vi "Simple UDP - Sender.vi"(8 "Stop":bool, 11 "Hand Coord.":dbl[](array[numeric])=[1000.0, 1000.0, 1000.0]) -> ()   [LabVIEW 2017]
doc: "The UDP protocol differs from TCP in that there is no error-checking with the packets of information that are sent, and thus no guarantee whatsoever that an intended recipient will actually receive a given piece of data.\n\nUDP does offer the ability to \"broadcast\" data across a network--simply specify an IP Address of all ones (255.255.255.255) to attempt to broadcast information network-wide. Keep in mind that routers and other network hardware will generally refuse to forward the broadcast beyond certain points, so the extent of the broadcast will in practice be limited."
panel:
  out "concatenated string output":string
  out "normalized x 100":dbl[](array[numeric])
  # "Overview: Demonstrates the use of the UDP functions to send data over a UDP connection.\nInstructions:\n1. Run the VI.\n2. Open Simple UDP - Receiver.vi and follow the instructions on its front panel.\n3. Click Stop to stop the VI."
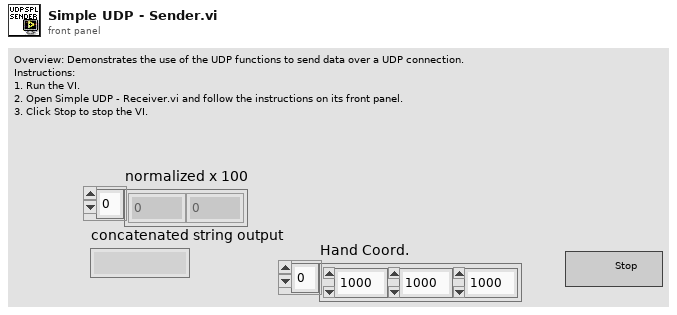
[diagram p1: front panel]
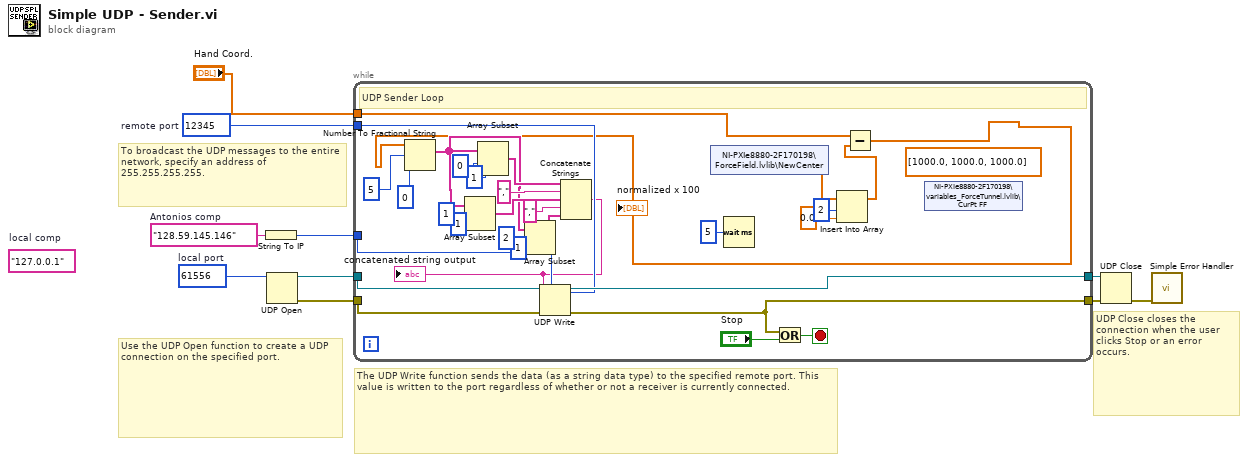
[diagram p0: block diagram]
diagram:
  (unwired) "127.0.0.1"  # local comp
  w2 = u16 12345  # remote port
  w3 = u16 61556  # local port
  w8 = "128.59.145.146"  # Antonios comp
  # "To broadcast the UDP messages to the entire network, specify an address of 255.255.255.255."
  # "UDP Close closes the connection when the user clicks Stop or an error occurs."
  # "The UDP Write function sends the data (as a string data type) to the specified remote port. This value is written to the port regardless of whether or not a receiver is currently connected."
  # "Use the UDP Open function to create a UDP connection on the specified port."
  n1 = String To IP(1:w8) -> (0:w6:u32)
  n2 = UDP Open(11:w3) -> (port=w5:refnum<k16>, 0:w4:errorcluster)  [unwired: 4 in, 1 out]
  n3 = while {
    tunnel: [w35] -> w9
    tunnel: w5 -> [w40]
    tunnel: w4 -> [w39]
    tunnel: [w36] -> w10
    tunnel: w6 -> [w34]
    tunnel: w2 -> [w32]
    tunnel: "Hand Coord." -> [w11]
    stop <- w38 stop-if-true
    (unwired) dbl[] [1000.0, 1000.0, 1000.0] ("y")
    # "UDP Sender Loop"
    n4 = shared-variable "NI-PXIe8880-2F170198\\ForceField.lvlib\\NewCenter"() -> (w21:dbl[])  [unwired: 1 in, 1 out]
    n5 = Wait (ms)(milliseconds to wait=u32 5) -> ()  [unwired: 1 out]
    n6 = Insert Into Array(array=w21, index=2, new element=0.0 ("new element/subarray")) -> (w20:dbl[])
    n7 = Subtract(x=w11, y=w20) -> (x-y=w12:dbl[])
    "normalized x 100" <- w12
    n8 = Number To Fractional String(number=w12, width (-)=i16 5, precision (6)=i16 0) -> (F-format string=w14:string[])  [unwired: 1 in]
    n9 = Array Subset(array=w14, index=1, length=1) -> (w25:string[])
    n10 = Array Subset(array=w14, index=0, length=1) -> (w29:string[])
    n11 = Array Subset(array=w14, index=2, length=1) -> (w13:string[])
    n12 = Concatenate Strings(w29, ",", w25, ",", w13) -> (w28:string)
    "concatenated string output" <- w28
    n13 = UDP Write(address=w34, port or service name=w32, connection ID=w40, data in=w28, 8:w39) -> (error out=w35:errorcluster, 3:w36:refnum<k16>)  [unwired: 1 in]
    n14 = Or(x=w35, y="Stop") -> (x .or. y?=w38:bool)
    n15 = shared-variable "NI-PXIe8880-2F170198\\variables_ForceTunnel.lvlib\\CurPt FF"() -> ()  [unwired: 1 in, 2 out]
  }
  n16 = UDP Close(connection ID=w10, 8:w9) -> (error out=w7:errorcluster)  [unwired: 1 out]
  n17 = call <vilib>:"Simple Error Handler.vi"("error in (no error)"=w7) -> ()  [unwired: 4 in, 5 out]
